vi "IEEE_754.vi"() -> ()   [LabVIEW 2015]
panel:
  out "Exponent":string
  out "Mantissa":string
  out "Sign":string
  out "2진수":u32 format="%b"
  in  "문자열":string
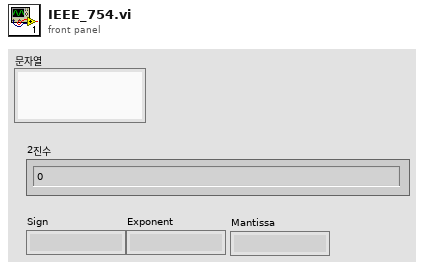
[diagram p1: front panel]
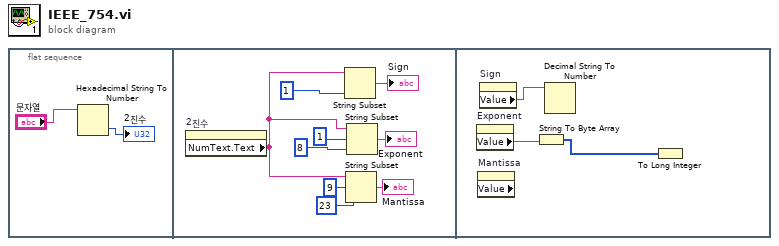
[diagram p0: block diagram]
diagram:
  n1 = flat-sequence {
    frame #0 {
      n2 = Hexadecimal String To Number(string="문자열") -> (number=→"2진수":u32)  [unwired: 2 in, 1 out]
    }
    frame #1 {
      n3 = property on="2진수" class="DigNum (엄격한)"() -> ("NumText.Text"=w9:string)  [unwired: 2 in, 2 out]
      n4 = String Subset(string=w9, length (rest)=1 ("길이(나머지)")) -> (substring=→"Sign":string)  [unwired: 1 in]
      n5 = String Subset(string=w9, offset (0)=9 ("오프셋(0)"), length (rest)=23 ("길이(나머지)")) -> (substring=→"Mantissa":string)
      n6 = String Subset(string=w9, offset (0)=1 ("오프셋(0)"), length (rest)=8 ("길이(나머지)")) -> (substring=→"Exponent":string)
    }
    frame #2 {
      n7 = property on="Exponent" class="Str"() -> ("Value"=w13:string)  [unwired: 2 in, 2 out]
      n8 = property on="Mantissa" class="Str" props=["Value"]() -> ()  [unwired: 2 in, 3 out]
      n9 = property on="Sign" class="Str"() -> ("Value"=w14:string)  [unwired: 2 in, 2 out]
      n10 = String To Byte Array(string=w13) -> (unsigned byte array=w12:u8[])
      n11 = Decimal String To Number(string=w14) -> ()  [unwired: 2 in, 2 out]
      n12 = To Long Integer(number=w12) -> ()  [unwired: 1 out]
    }
  }
